vi "Convert CLFN Element to LabVIEW Element.vi"(5 "Converter Owner":refnum<vi>, 9 "Element Sink Terminal":refnum<vi>, 10 "Element Source Terminal":refnum<vi>, 11 "Abstract Param Writer In":refnum<class "Abstract Param Writer.lvclass">) -> (3 "Abstract Param Writer Out":refnum<class "Abstract Param Writer.lvclass">)   [LabVIEW 2013, in "Abstract Param Writer.lvclass"]
uses:
  Abstract Param Writer.lvclass
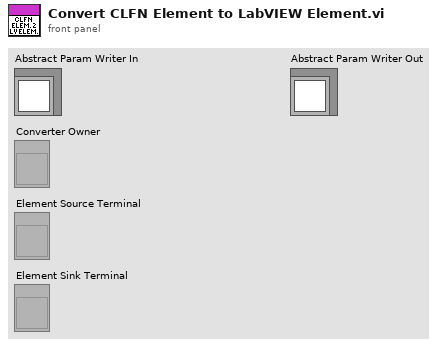
[diagram p1: front panel]
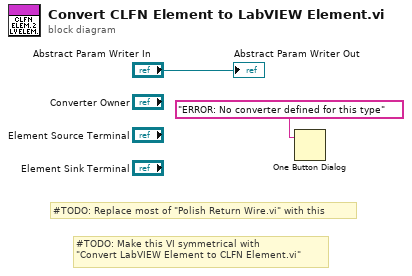
[diagram p0: block diagram]
diagram:
  # "#TODO: Make this VI symmetrical with\n\"Convert LabVIEW Element to CLFN Element.vi\""
  # "#TODO: Replace most of \"Polish Return Wire.vi\" with this"
  n1 = One Button Dialog(message="ERROR: No converter defined for this type") -> ()  [unwired: 1 in, 1 out]
  "Abstract Param Writer Out" <- "Abstract Param Writer In"
